vi "TempAlgoTest (SubVI).vi"(0 "Temp":refnum<vi>, 1 "Speed Ind":dbl format="%#_13g", 2 "Motor Speed RPM":refnum<vi>, 3 "Round":T1(ring), 4 "Temp Up In":dbl format="%#_13g", 5 "error in (no error)":errorcluster, 6 "String in":refnum<vi>, 7 "Temp Goal":dbl format="%#_13g", 8 "Stop":refnum<vi>, 9 "Speed Goal":dbl format="%#_13g", 10 "Stop BurnIn":refnum<vi>, 12 "Strin":string) -> (14 "Speed Pass/Fail":bool, 15 "Temp  Pass/Fail":dbl, 16 "Temp Up Out":dbl, 17 "Speed Pass/Fail":dbl, 18 "Temp Pass/Fail":bool, 19 "error out":errorcluster)   [LabVIEW 2017]
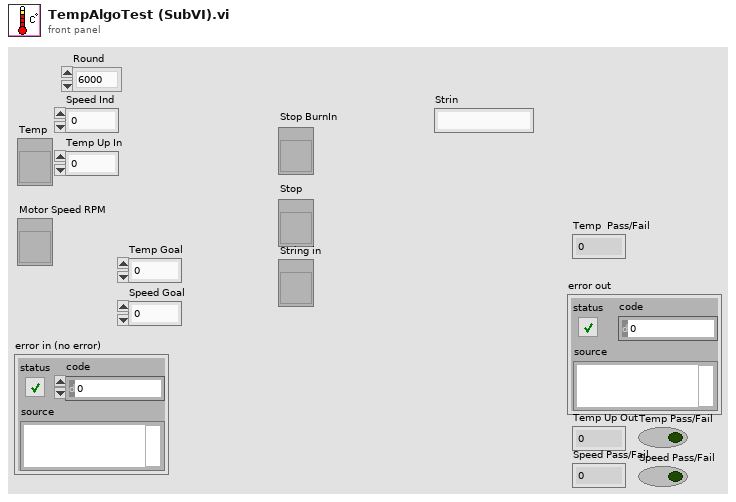
[diagram p1: front panel]
types:
  T1 = enum32{"6000", "11500", "15100", "11500-2", "6000-2"}
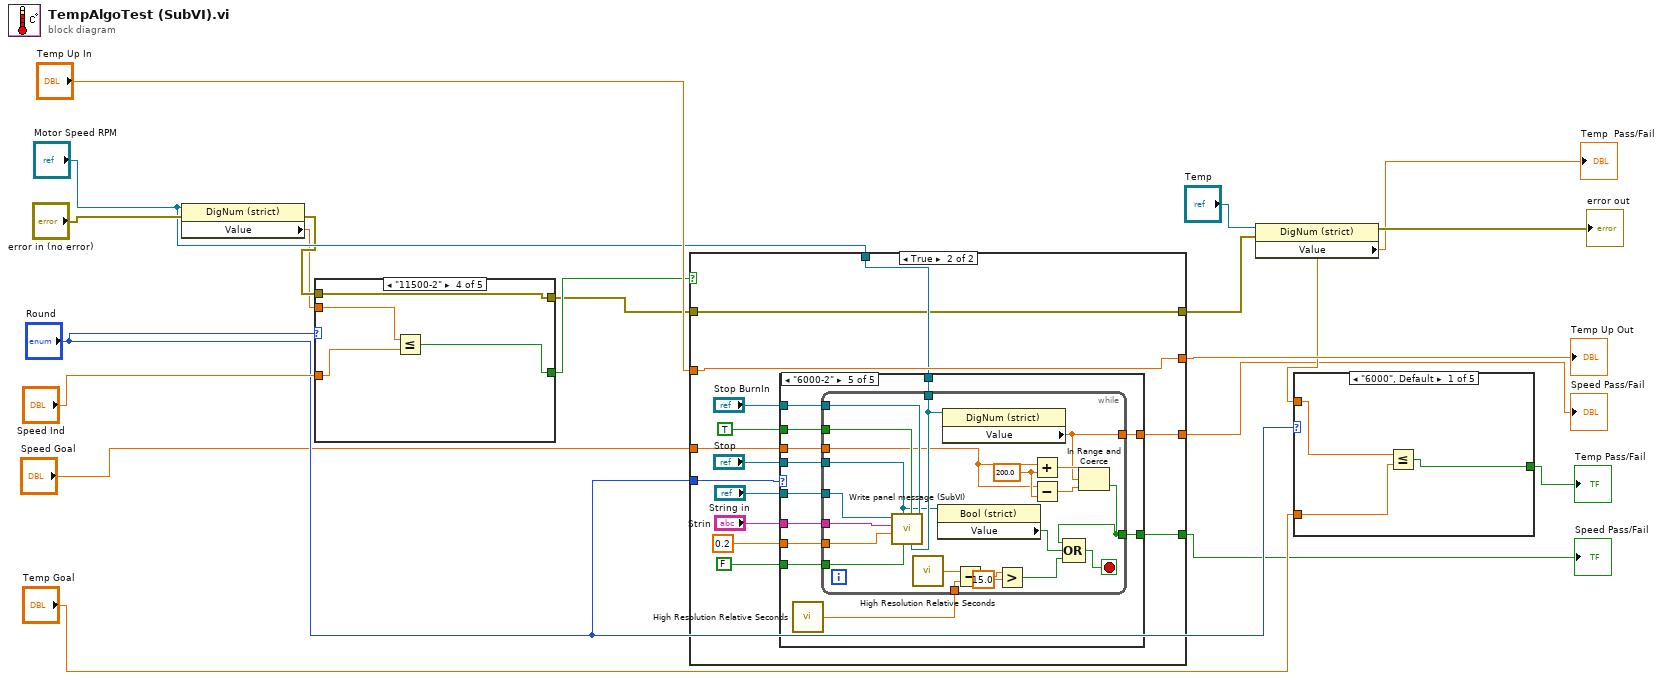
[diagram p0: block diagram]
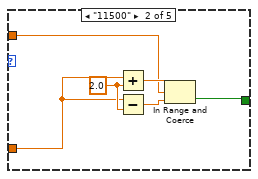
[diagram p2: hidden frame]
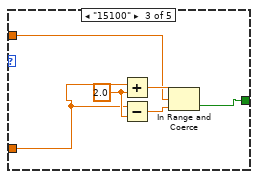
[diagram p3: hidden frame]
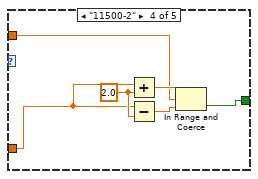
[diagram p4: hidden frame]
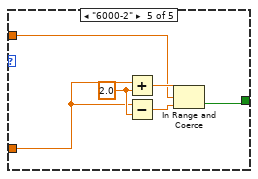
[diagram p5: hidden frame]
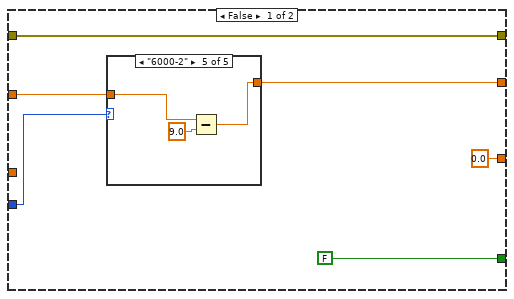
[diagram p6: hidden frame]
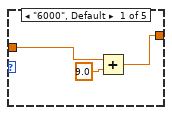
[diagram p7: hidden frame]
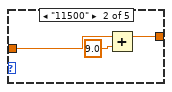
[diagram p8: hidden frame]
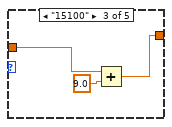
[diagram p9: hidden frame]
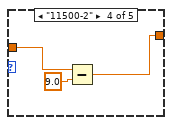
[diagram p10: hidden frame]
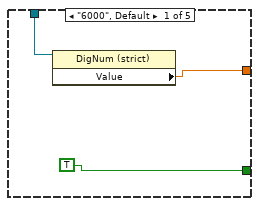
[diagram p11: hidden frame]
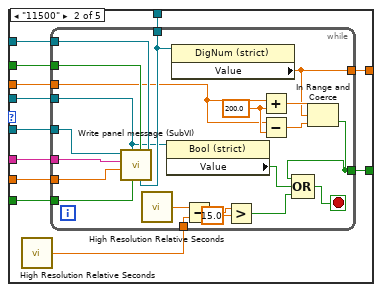
[diagram p12: hidden frame]
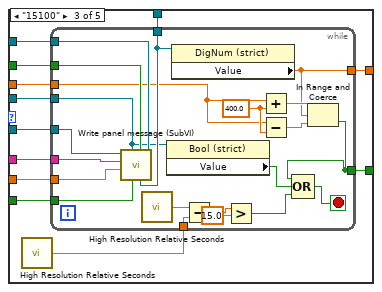
[diagram p13: hidden frame]
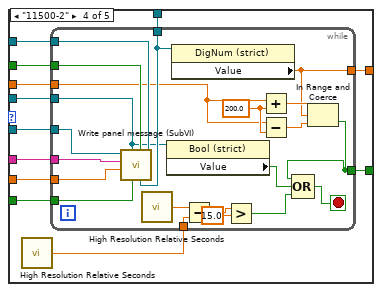
[diagram p14: hidden frame]
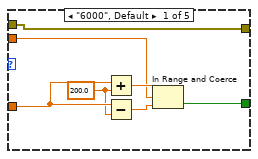
[diagram p15: hidden frame]
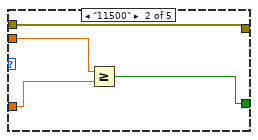
[diagram p16: hidden frame]
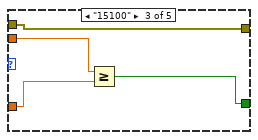
[diagram p17: hidden frame]
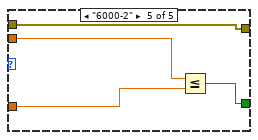
[diagram p18: hidden frame]
diagram:
  n1 = property class="DigNum (strict)"(reference="Motor Speed RPM", error in="error in (no error)") -> (error out=w6:errorcluster, "Value"=w3:dbl)  [unwired: 1 out]
  n2 = case shown="\"11500-2\"" "Round" {
    tunnel: w3 -> [w23 w30 w34 w38 w42]
    tunnel: "Speed Ind" -> [w24 w29 w33 w37 w41]
    tunnel: [w21 w28 w32 w36 w40] -> w14
    tunnel: w6 -> [w20 w27 w31 w35 w39]
    tunnel: [w20 w27 w31 w35 w39] -> w5
    frame "6000", Default {
      w22 = 200.0 ("y")
      n3 = Add(x=w24, y=w22) -> (x+y=w26:dbl)
      n4 = Subtract(x=w24, y=w22) -> (x-y=w25:dbl)
      n5 = In Range and Coerce(upper limit=w26, x=w23, lower limit=w25) -> (In Range?=w21:bool)  [unwired: 1 out]
    }
    frame "11500" {
      n6 = Greater Or Equal?(x=w30, y=w29) -> (x >= y?=w28:bool)
    }
    frame "15100" {
      n7 = Greater Or Equal?(x=w34, y=w33) -> (x >= y?=w32:bool)
    }
    frame "11500-2" {
      n8 = Less Or Equal?(x=w38, y=w37) -> (x <= y?=w36:bool)
    }
    frame "6000-2" {
      n9 = Less Or Equal?(x=w42, y=w41) -> (x <= y?=w40:bool)
    }
  }
  n10 = case shown="True" w14 {
    tunnel: "Temp Up In" -> [w48 w77]
    tunnel: [w47 w77] -> w13
    tunnel: "Motor Speed RPM" -> [_ w69]
    tunnel: "Round" -> [w43 w68]
    tunnel: [FALSE ("rpm 2") w67] -> w7
    tunnel: w5 -> [w45 w66]
    tunnel: [w45 w66] -> w4
    tunnel: "Speed Goal" -> [_ w65]
    tunnel: [0.0 ("Value") w64] -> w1
    frame False {
      n11 = case shown="\"6000-2\"" w43 {
        tunnel: w48 -> [w50 w54 w56 w59 w62]
        tunnel: [w49 w52 w55 w58 w61] -> w47
        frame "6000", Default {
          n12 = Add(x=w50, y=9.0) -> (x+y=w49:dbl)
        }
        frame "11500" {
          n13 = Add(x=w54, y=9.0) -> (x+y=w52:dbl)
        }
        frame "15100" {
          n14 = Add(x=w56, y=9.0) -> (x+y=w55:dbl)
        }
        frame "11500-2" {
          n15 = Subtract(x=w59, y=9.0) -> (x-y=w58:dbl)
        }
        frame "6000-2" {
          n16 = Subtract(x=w62, y=9.0) -> (x-y=w61:dbl)
        }
      }
    }
    frame True {
      n17 = case shown="\"6000-2\"" w68 {
        tunnel: "Stop BurnIn" -> [_ w92 w125 w158 w191]
        tunnel: TRUE ("rpm 2") -> [_ w91 w124 w157 w190]
        tunnel: FALSE ("PrintTime") -> [_ w90 w123 w156 w189]
        tunnel: "Stop" -> [_ w89 w122 w155 w188]
        tunnel: 0.2 ("Time to wait") -> [_ w88 w121 w154 w187]
        tunnel: "Strin" -> [_ w87 w120 w153 w186]
        tunnel: "String in" -> [_ w86 w119 w152 w185]
        tunnel: w69 -> [w79 w85 w118 w151 w184]
        tunnel: [TRUE ("rpm 2") w82 w115 w148 w181] -> w67
        tunnel: w65 -> [_ w84 w117 w150 w183]
        tunnel: [w78 w83 w116 w149 w182] -> w64
        frame "6000", Default {
          n18 = property class="DigNum (strict)"(reference=w79) -> ("Value"=w78:dbl)  [unwired: 1 in, 2 out]
        }
        frame "11500" {
          n19 = call <vilib>:"High Resolution Relative Seconds.vi"() -> ("relative seconds"=w81:dbl)
          n20 = while {
            tunnel: w92 -> [w113]
            tunnel: w91 -> [w112]
            tunnel: w90 -> [w111]
            tunnel: w89 -> [w106]
            tunnel: w88 -> [w110]
            tunnel: w87 -> [w109]
            tunnel: w86 -> [w108]
            tunnel: w85 -> [w107]
            tunnel: w84 -> [w102]
            tunnel: [w101] -> w83
            tunnel: [w99] -> w82
            tunnel: w81 -> [w96]
            stop <- w100 stop-if-true
            w105 = 200.0 ("y")
            n21 = call "Write panel message (SubVI).vi"("Stop BurnIn"=w113, 4:"rpm"=w107, 5:"rpm"=w112, "PrintTime"=w111, "Stop"=w106, "Time to wait"=w110, "Strin"=w109, "String in"=w108) -> ()  [unwired: 3 in, 1 out]
            n22 = call <vilib>:"High Resolution Relative Seconds.vi"() -> ("relative seconds"=w97:dbl)
            n23 = property class="Bool (strict)"(reference=w106) -> ("Value"=w98:bool)  [unwired: 1 in, 2 out]
            n24 = property class="DigNum (strict)"(reference=w107) -> ("Value"=w101:dbl)  [unwired: 1 in, 2 out]
            n25 = Subtract(x=w97, y=w96) -> (x-y=w95:dbl)
            n26 = Greater?(x=w95, y=15.0) -> (0:w93:bool)
            n27 = Add(x=w102, y=w105) -> (x+y=w103:dbl)
            n28 = Subtract(x=w102, y=w105) -> (x-y=w104:dbl)
            n29 = In Range and Coerce(upper limit=w103, x=w101, lower limit=w104) -> (In Range?=w99:bool)  [unwired: 1 out]
            n30 = Compound Arithmetic op=OR(w99, w98, w93) -> (w100:bool)
          }
        }
        frame "15100" {
          n31 = call <vilib>:"High Resolution Relative Seconds.vi"() -> ("relative seconds"=w114:dbl)
          n32 = while {
            tunnel: w125 -> [w146]
            tunnel: w124 -> [w145]
            tunnel: w123 -> [w144]
            tunnel: w122 -> [w139]
            tunnel: w121 -> [w143]
            tunnel: w120 -> [w142]
            tunnel: w119 -> [w141]
            tunnel: w118 -> [w140]
            tunnel: w117 -> [w135]
            tunnel: [w134] -> w116
            tunnel: [w132] -> w115
            tunnel: w114 -> [w129]
            stop <- w133 stop-if-true
            w138 = 400.0 ("y")
            n33 = call "Write panel message (SubVI).vi"("Stop BurnIn"=w146, 4:"rpm"=w140, 5:"rpm"=w145, "PrintTime"=w144, "Stop"=w139, "Time to wait"=w143, "Strin"=w142, "String in"=w141) -> ()  [unwired: 3 in, 1 out]
            n34 = call <vilib>:"High Resolution Relative Seconds.vi"() -> ("relative seconds"=w130:dbl)
            n35 = property class="Bool (strict)"(reference=w139) -> ("Value"=w131:bool)  [unwired: 1 in, 2 out]
            n36 = property class="DigNum (strict)"(reference=w140) -> ("Value"=w134:dbl)  [unwired: 1 in, 2 out]
            n37 = Subtract(x=w130, y=w129) -> (x-y=w128:dbl)
            n38 = Greater?(x=w128, y=15.0) -> (0:w126:bool)
            n39 = Add(x=w135, y=w138) -> (x+y=w136:dbl)
            n40 = Subtract(x=w135, y=w138) -> (x-y=w137:dbl)
            n41 = In Range and Coerce(upper limit=w136, x=w134, lower limit=w137) -> (In Range?=w132:bool)  [unwired: 1 out]
            n42 = Compound Arithmetic op=OR(w132, w131, w126) -> (w133:bool)
          }
        }
        frame "11500-2" {
          n43 = call <vilib>:"High Resolution Relative Seconds.vi"() -> ("relative seconds"=w147:dbl)
          n44 = while {
            tunnel: w158 -> [w179]
            tunnel: w157 -> [w178]
            tunnel: w156 -> [w177]
            tunnel: w155 -> [w172]
            tunnel: w154 -> [w176]
            tunnel: w153 -> [w175]
            tunnel: w152 -> [w174]
            tunnel: w151 -> [w173]
            tunnel: w150 -> [w168]
            tunnel: [w167] -> w149
            tunnel: [w165] -> w148
            tunnel: w147 -> [w162]
            stop <- w166 stop-if-true
            w171 = 200.0 ("y")
            n45 = call "Write panel message (SubVI).vi"("Stop BurnIn"=w179, 4:"rpm"=w173, 5:"rpm"=w178, "PrintTime"=w177, "Stop"=w172, "Time to wait"=w176, "Strin"=w175, "String in"=w174) -> ()  [unwired: 3 in, 1 out]
            n46 = call <vilib>:"High Resolution Relative Seconds.vi"() -> ("relative seconds"=w163:dbl)
            n47 = property class="Bool (strict)"(reference=w172) -> ("Value"=w164:bool)  [unwired: 1 in, 2 out]
            n48 = property class="DigNum (strict)"(reference=w173) -> ("Value"=w167:dbl)  [unwired: 1 in, 2 out]
            n49 = Subtract(x=w163, y=w162) -> (x-y=w161:dbl)
            n50 = Greater?(x=w161, y=15.0) -> (0:w159:bool)
            n51 = Add(x=w168, y=w171) -> (x+y=w169:dbl)
            n52 = Subtract(x=w168, y=w171) -> (x-y=w170:dbl)
            n53 = In Range and Coerce(upper limit=w169, x=w167, lower limit=w170) -> (In Range?=w165:bool)  [unwired: 1 out]
            n54 = Compound Arithmetic op=OR(w165, w164, w159) -> (w166:bool)
          }
        }
        frame "6000-2" {
          n55 = call <vilib>:"High Resolution Relative Seconds.vi"() -> ("relative seconds"=w180:dbl)
          n56 = while {
            tunnel: w191 -> [w212]
            tunnel: w190 -> [w211]
            tunnel: w189 -> [w210]
            tunnel: w188 -> [w205]
            tunnel: w187 -> [w209]
            tunnel: w186 -> [w208]
            tunnel: w185 -> [w207]
            tunnel: w184 -> [w206]
            tunnel: w183 -> [w201]
            tunnel: [w200] -> w182
            tunnel: [w198] -> w181
            tunnel: w180 -> [w195]
            stop <- w199 stop-if-true
            w204 = 200.0 ("y")
            n57 = call "Write panel message (SubVI).vi"("Stop BurnIn"=w212, 4:"rpm"=w206, 5:"rpm"=w211, "PrintTime"=w210, "Stop"=w205, "Time to wait"=w209, "Strin"=w208, "String in"=w207) -> ()  [unwired: 3 in, 1 out]
            n58 = call <vilib>:"High Resolution Relative Seconds.vi"() -> ("relative seconds"=w196:dbl)
            n59 = property class="Bool (strict)"(reference=w205) -> ("Value"=w197:bool)  [unwired: 1 in, 2 out]
            n60 = property class="DigNum (strict)"(reference=w206) -> ("Value"=w200:dbl)  [unwired: 1 in, 2 out]
            n61 = Subtract(x=w196, y=w195) -> (x-y=w194:dbl)
            n62 = Greater?(x=w194, y=15.0) -> (0:w192:bool)
            n63 = Add(x=w201, y=w204) -> (x+y=w202:dbl)
            n64 = Subtract(x=w201, y=w204) -> (x-y=w203:dbl)
            n65 = In Range and Coerce(upper limit=w202, x=w200, lower limit=w203) -> (In Range?=w198:bool)  [unwired: 1 out]
            n66 = Compound Arithmetic op=OR(w198, w197, w192) -> (w199:bool)
          }
        }
      }
    }
  }
  "Temp Up Out" <- w13
  "Speed Pass/Fail" <- w7
  "Speed Pass/Fail" <- w1
  n67 = property class="DigNum (strict)"(reference="Temp", error in=w4) -> (error out=→"error out":errorcluster, "Value"=w12:dbl)  [unwired: 1 out]
  "Temp  Pass/Fail" <- w12
  n68 = case shown="\"6000\", Default" "Round" {
    tunnel: w12 -> [w214 w218 w224 w230 w236]
    tunnel: [w215 w216 w222 w228 w234] -> w10
    tunnel: "Temp Goal" -> [w213 w217 w223 w229 w235]
    frame "6000", Default {
      n69 = Less Or Equal?(x=w214, y=w213) -> (x <= y?=w215:bool)
    }
    frame "11500" {
      w219 = 2.0 ("y")
      n70 = Add(x=w217, y=w219) -> (x+y=w221:dbl)
      n71 = Subtract(x=w217, y=w219) -> (x-y=w220:dbl)
      n72 = In Range and Coerce(upper limit=w221, x=w218, lower limit=w220) -> (In Range?=w216:bool)  [unwired: 1 out]
    }
    frame "15100" {
      w225 = 2.0 ("y")
      n73 = Add(x=w223, y=w225) -> (x+y=w227:dbl)
      n74 = Subtract(x=w223, y=w225) -> (x-y=w226:dbl)
      n75 = In Range and Coerce(upper limit=w227, x=w224, lower limit=w226) -> (In Range?=w222:bool)  [unwired: 1 out]
    }
    frame "11500-2" {
      w231 = 2.0 ("y")
      n76 = Add(x=w229, y=w231) -> (x+y=w233:dbl)
      n77 = Subtract(x=w229, y=w231) -> (x-y=w232:dbl)
      n78 = In Range and Coerce(upper limit=w233, x=w230, lower limit=w232) -> (In Range?=w228:bool)  [unwired: 1 out]
    }
    frame "6000-2" {
      w237 = 2.0 ("y")
      n79 = Add(x=w235, y=w237) -> (x+y=w239:dbl)
      n80 = Subtract(x=w235, y=w237) -> (x-y=w238:dbl)
      n81 = In Range and Coerce(upper limit=w239, x=w236, lower limit=w238) -> (In Range?=w234:bool)  [unwired: 1 out]
    }
  }
  "Temp Pass/Fail" <- w10
